vi "acout.vi"() -> ()   [LabVIEW 2010]
doc: "I. Description:\nThis example demonstrates how to take a single Measurement (Sample) from an Analog Input Channel.\n\nII. Instructions for Running:\n1. Select the Physical Channel to correspond to where your signal is input on the DAQ device.\n2. Enter the Minimum and Maximum Voltage Ranges\nNote: For better accuracy try to match the Input Ranges to the expected voltage level of the measured signal.\nNote: Use the Gen Voltage Update example to provide a signal on your DAQ device to measure.\n\nIII. Block Diagram Steps:\n1. Create an Analog Input Voltage Channel.\n2. Use the Read VI to Measure 1 Sample from 1 Channel on the Data\nAcquisition Card. Set a timeout so an error is returned if the sample\nis not returned in the specified time limit\n3. Call the Clear Task VI to clear the Task.\n4. Use the popup dialog box to display an error if any.\n\nIV. I/O Connections Overview:\nMake sure your signal input terminal matches the Physical Channel I/O Control."
uses:
  <vilib>/Utility/error.llb/DialogType.ctl
  <vilib>/DAQmx/write.llb/DAQmx Write (Analog Wfm 1Chan NSamp).vi
  <vilib>/DAQmx/read.llb/DAQmx Read (Analog Wfm 1Chan NSamp).vi
  <vilib>/DAQmx/create/channels.llb/DAQmx Create Channel (AI-Voltage-Basic).vi
  <vilib>/DAQmx/create/channels.llb/DAQmx Create Channel (AO-Voltage-Basic).vi
  <vilib>/Utility/file.llb/Write To Spreadsheet File (DBL).vi
  <vilib>/measure/mascope.llb/Amplitude and Levels 1 chan.vi
  <vilib>/measure/madcrms.llb/Basic Averaged DC-RMS for 1 Chan.vi
  <vilib>/daqmx/miscellaneous.llb/DAQmx Fill In Error Info.vi
  <vilib>/measure/NI_MAPro.lvlib
panel:
  out "Waveform Entrada":waveform(dbl)(graph)
  out "Waveform Medida":waveform(dbl)(graph)
  in  "Duracion (s)":dbl=-10.0 format="%0.2f"
  in  "Amplitud":dbl=-10.0 format="%0.2f"
  out "Vez #":i32
  out "Paso #":i32
  in  "Freq Paso":dbl step=0.001 format="%0.3f"
  in  "Freq Hasta":dbl step=0.001 format="%0.3f"
  in  "Freq Desde":dbl step=0.001 format="%0.3f"
  out "Numeric":u32
  in  "Corre":bool
  in  "Maximum Value 2":dbl=10.0 caption="Maximum Value" format="%.2f"
  in  "Minimum Value 2":dbl=-10.0 caption="Minimum Value" format="%0.2f"
  out "In Range?":bool
  in  "Physical Channel 2":tag="Dev1/ai0" caption="Physical Channel"
  in  "stop":bool
  in  "Maximum Value":dbl=10.0 format="%.2f"
  in  "Minimum Value":dbl=-10.0 format="%0.2f"
  in  "Physical Channel":tag="Dev1/ai0"
  # "Channel Parameters"
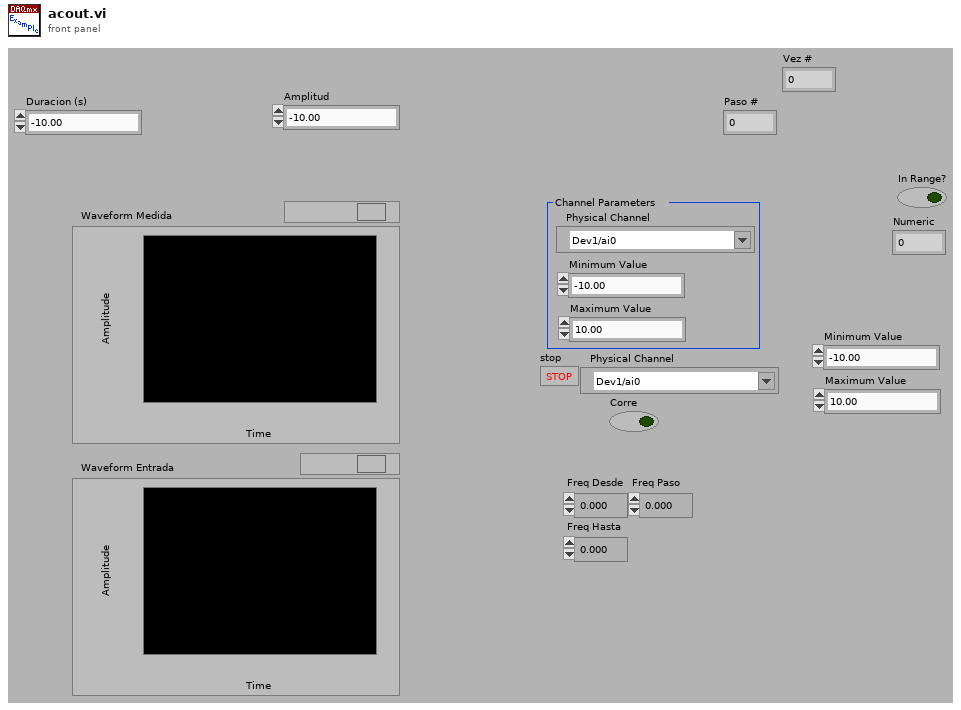
[diagram p1: front panel]
types:
  T1 = typedef "DialogType.ctl" = u16
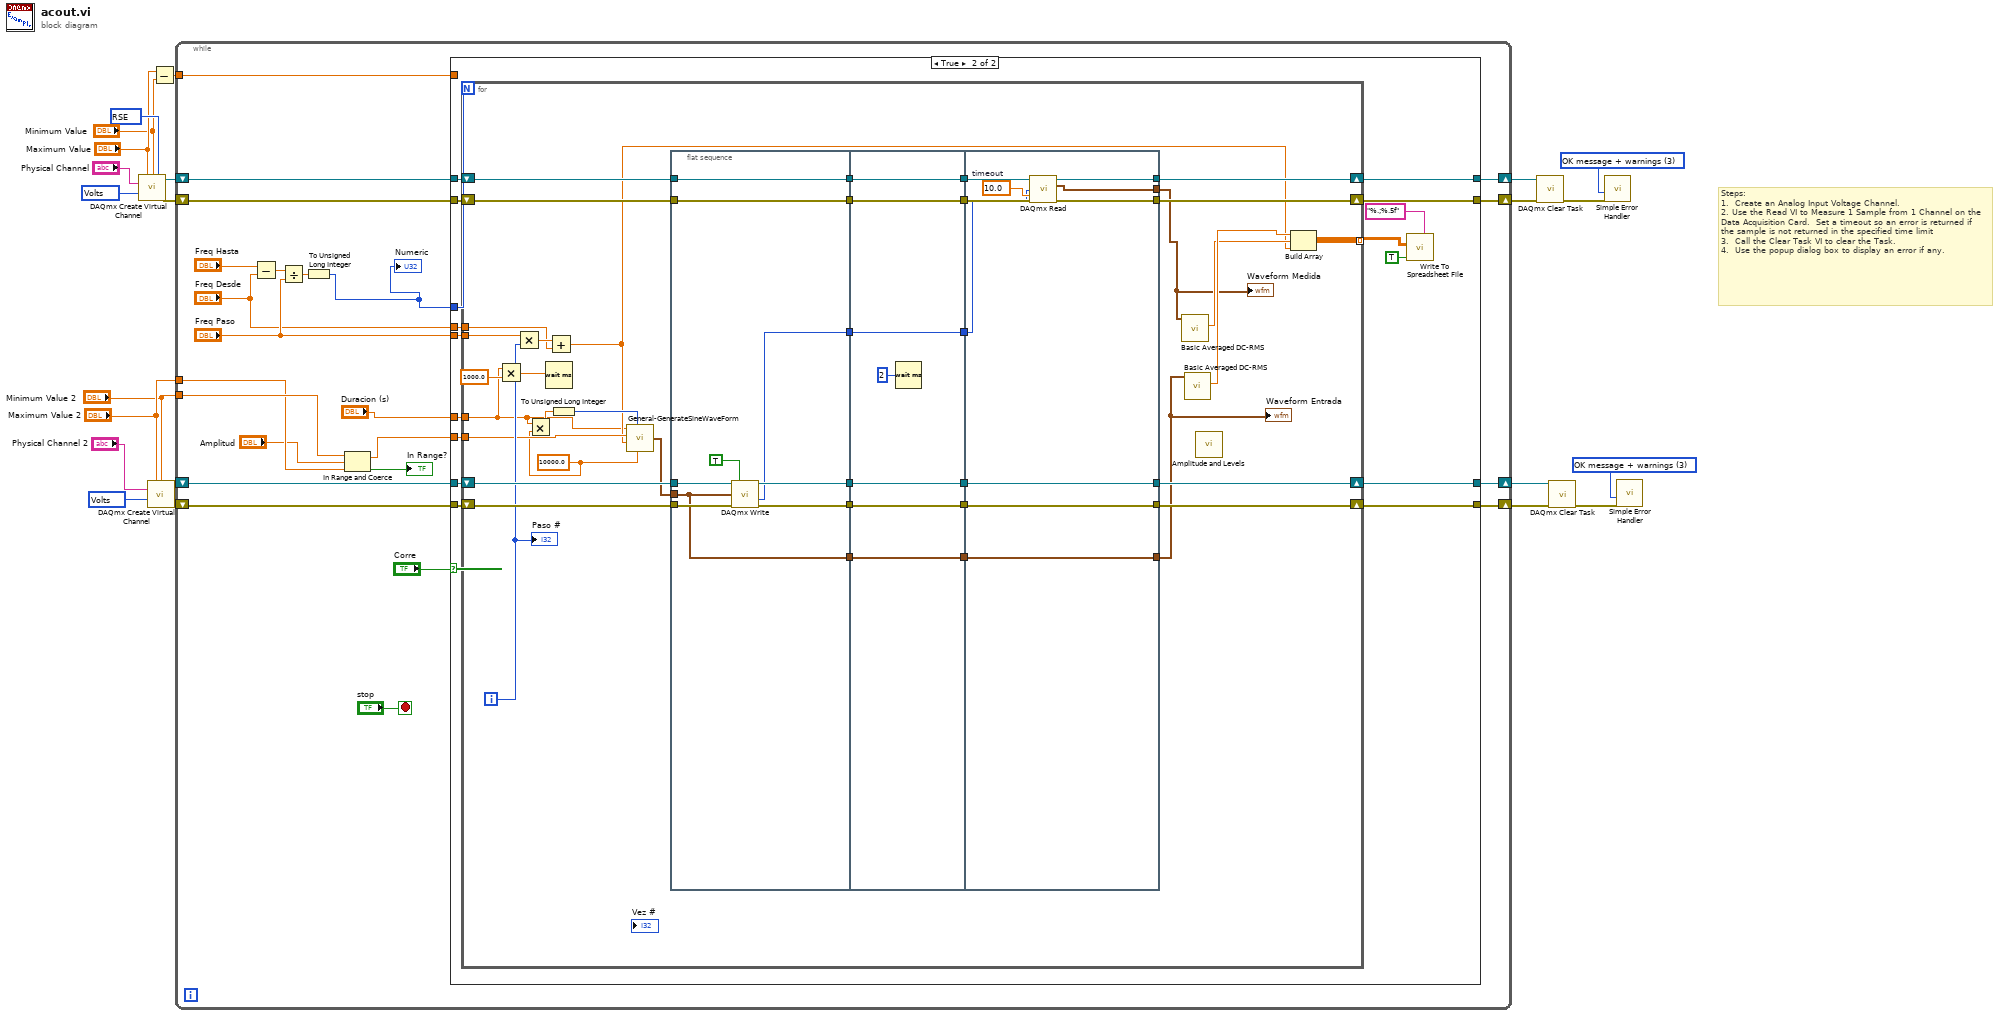
[diagram p0: block diagram]
diagram:
  w6 = 10083 items=["default"=-1, "RSE"=10083, "NRSE"=10078, "Differential"=10106, "Pseudodifferential"=12529] ("input terminal configuration")
  w7 = 10348 items=["Volts"=10348, "From Custom Scale"=10065] ("units")
  w8 = 10348 items=["Volts"=10348, "From Custom Scale"=10065] ("units")
  w12 = T1 3 items=["no dialog", "OK message", "continue or stop message", "OK message + warnings", "continue/stop + warnings"] ("type of dialog (OK msg:1)")
  w19 = T1 3 items=["no dialog", "OK message", "continue or stop message", "OK message + warnings", "continue/stop + warnings"] ("type of dialog (OK msg:1)")
  # "Steps: \n1.  Create an Analog Input Voltage Channel. \n2. Use the Read VI to Measure 1 Sample from 1 Channel on the Data Acquisition Card.  Set a timeout so an error is returned if the sample is not returned in the specified time limit\n3.  Call the Clear Task VI to clear the Task.\n4.  Use the popup dialog box to display an error if any."
  n1 = call-poly <vilib>:"DAQmx Create Virtual Channel.vi"("maximum value"="Maximum Value", "minimum value"="Minimum Value", "input terminal configuration"=w6, "physical channels"="Physical Channel", "units"=w8) -> ("task out"=w21:refnum<k21>, "error out"=w20:errorcluster)  [unwired: 9 in]
  n2 = call-poly <vilib>:"DAQmx Create Virtual Channel.vi"("maximum value"="Maximum Value 2", "minimum value"="Minimum Value 2", "physical channels"="Physical Channel 2", "units"=w7) -> ("task out"=w14:refnum<k21>, "error out"=w13:errorcluster)  [unwired: 10 in]
  n3 = Subtract(x="Maximum Value", y="Minimum Value") -> (x-y=w1:dbl)
  n4 = while {
    shift-right: [w39] -> w18
    shift-left: w21 -> [w42]
    shift-right: [w40] -> w17
    shift-left: w20 -> [w41]
    shift-right: [w38] -> w10
    shift-left: w14 -> [w44]
    shift-right: [w37] -> w9
    shift-left: w13 -> [w43]
    tunnel: "Maximum Value 2" -> [w26]
    tunnel: "Minimum Value 2" -> [w27]
    tunnel: w1 -> [w30]
    stop <- "stop" stop-if-true
    n5 = Subtract(x="Freq Hasta", y="Freq Desde") -> (x-y=w34:dbl)
    n6 = Divide(x=w34, y="Freq Paso") -> (x/y=w33:dbl)
    n7 = To Unsigned Long Integer(number=w33) -> (unsigned 32bit integer=w29:u32)
    "Numeric" <- w29
    n8 = In Range and Coerce(upper limit=w27, x="Amplitud", lower limit=w26) -> (coerced(x)=w24:dbl, In Range?=→"In Range?":bool)
    n9 = case shown="True" "Corre" {
      tunnel: w44 -> [w47 w65]
      tunnel: w43 -> [w46 w64]
      tunnel: w42 -> [w49 w63]
      tunnel: w41 -> [w48 w62]
      tunnel: [w48 w61] -> w40
      tunnel: [w49 w60] -> w39
      tunnel: [w47 w59] -> w38
      tunnel: [w46 w58] -> w37
      tunnel: w29 -> [_ w57]
      tunnel: "Freq Paso" -> [_ w56]
      tunnel: "Freq Desde" -> [_ w55]
      tunnel: w30 -> [_ _]
      tunnel: w24 -> [_ w51]
      tunnel: "Duracion (s)" -> [_ w50]
      frame False {
      }
      frame True {
        n10 = for {
          N: w57 -> [_]
          shift-right: [w99] -> w61
          shift-left: w62 -> [w100]
          shift-right: [w98] -> w60
          shift-left: w63 -> [w101]
          shift-right: [w97] -> w59
          shift-left: w65 -> [w103]
          shift-right: [w96] -> w58
          shift-left: w64 -> [w102]
          tunnel: w56 -> [w94]
          tunnel: w55 -> [w93]
          tunnel: [w92] -> w54 mode=indexing
          tunnel: w51 -> [w82]
          tunnel: w50 -> [w66]
          i -> [w91]
          w81 = 10000.0 ("Fs (S/s)")
          n11 = Multiply(x=w66, y=1000.0) -> (x*y=w68:dbl)
          n12 = Multiply(x=w94, y=w91) -> (x*y=w95:dbl)
          n13 = Multiply(x=w66, y=w81) -> (x*y=w79:dbl)
          n14 = Wait (ms)(milliseconds to wait=w68) -> ()  [unwired: 1 out]
          n15 = Add(x=w95, y=w93) -> (x+y=w73:dbl)
          n16 = To Unsigned Long Integer(number=w79) -> (unsigned 32bit integer=w80:u32)
          n17 = call "General-GenerateSineWaveForm.vi"("tiempo (s)"=w66, "#samples"=w80, "Amplitud"=w82, "frecuencia"=w73, "Fs (S/s)"=w81) -> ("Waveform"=w78:waveform(dbl))  [unwired: 3 in]
          n18 = flat-sequence {
            tunnel: w103 -> [w110]
            tunnel: w102 -> [w109]
            tunnel: [w112] -> w90
            tunnel: w101 -> [w112]
            tunnel: w100 -> [w111]
            tunnel: [w111] -> w89
            tunnel: [w108] -> w88
            tunnel: [w107] -> w87
            tunnel: w78 -> [w105]
            tunnel: [w105] -> w76
            tunnel: [w104] -> w72
            tunnel: w90 -> [w119]
            tunnel: [w119] -> w86
            tunnel: w89 -> [w118]
            tunnel: [w118] -> w85
            tunnel: w88 -> [w117]
            tunnel: [w117] -> w84
            tunnel: w87 -> [w116]
            tunnel: [w116] -> w83
            tunnel: [w114] -> w77
            tunnel: w76 -> [w114]
            tunnel: w72 -> [w113]
            tunnel: [w113] -> w71
            tunnel: w86 -> [w128]
            tunnel: w85 -> [w127]
            tunnel: [w126] -> w99
            tunnel: [w125] -> w98
            tunnel: w84 -> [w124]
            tunnel: [w124] -> w97
            tunnel: w83 -> [w123]
            tunnel: [w123] -> w96
            tunnel: [w122] -> w70
            tunnel: [w121] -> w69
            tunnel: w77 -> [w121]
            tunnel: w71 -> [w120]
            frame #0 {
              n19 = call-poly <vilib>:"DAQmx Write.vi"("task/channels in"=w110, "auto start"=TRUE, "data"=w105, "error in"=w109) -> ("task out"=w108:refnum<k21>, "number of samples written per channel"=w104:u32, "error out"=w107:errorcluster)  [unwired: 9 in]
            }
            frame #1 {
              n20 = Wait (ms)(milliseconds to wait=u32 2) -> ()  [unwired: 1 out]
            }
            frame #2 {
              w129 = 10.0  # timeout
              n21 = call-poly <vilib>:"DAQmx Read.vi"("task/channels in"=w128, "number of samples per channel"=w120, "timeout"=w129, "error in"=w127) -> ("task out"=w125:refnum<k21>, "data"=w122:waveform(dbl), "error out"=w126:errorcluster)  [unwired: 9 in]
            }
          }
          n22 = call-poly <vilib>:"Basic Averaged DC-RMS.vi"("signal in"=w70) -> ("RMS value"=w74:dbl)  [unwired: 7 in, 3 out]
          n23 = call-poly <vilib>:"Basic Averaged DC-RMS.vi"("signal in"=w69) -> ("RMS value"=w75:dbl)  [unwired: 7 in, 3 out]
          n24 = call-poly <vilib>:"Amplitude and Levels.vi"() -> ()  [unwired: 8 in, 4 out]
          n25 = Build Array(w75, w74, w73) -> (w92:dbl[])
          "Paso #" <- w91
          "Waveform Medida" <- w70
          "Waveform Entrada" <- w69
        }
        n26 = call-poly <vilib>:"Write To Spreadsheet File.vi"("format (%.3f)"="%.;%.5f", "append to file? (new file:F)"=TRUE, "2D data"=w54) -> ()  [unwired: 5 in, 1 out]
      }
    }
  }
  n27 = call <vilib>:"DAQmx Clear Task.vi"("task in"=w18, "error in"=w17) -> ("error out"=w16:errorcluster)  [unwired: 13 in]
  n28 = call <vilib>:"DAQmx Clear Task.vi"("task in"=w10, "error in"=w9) -> ("error out"=w11:errorcluster)  [unwired: 13 in]
  n29 = call <vilib>:"Simple Error Handler.vi"("type of dialog (OK msg:1)"=w19, "error in (no error)"=w16) -> ()  [unwired: 3 in, 5 out]
  n30 = call <vilib>:"Simple Error Handler.vi"("type of dialog (OK msg:1)"=w12, "error in (no error)"=w11) -> ()  [unwired: 3 in, 5 out]
